vi "Reset.vi"(8 "error in (no error)":errorcluster, 11 "VISA resource name":refnum<visa-resource-name>) -> (0 "error out":errorcluster, 3 "VISA resource name out":refnum<visa-resource-name>)   [LabVIEW 2012]
doc: "Resets the instruments."
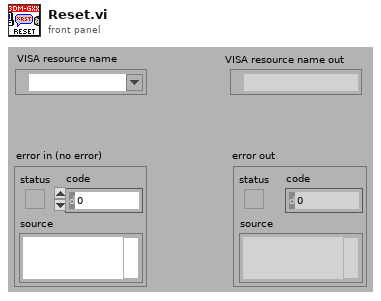
[diagram p1: front panel]
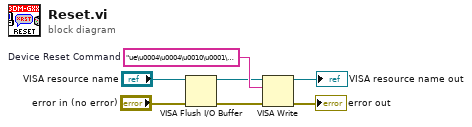
[diagram p0: block diagram]
diagram:
  w7 = "ue\u0004\u0004\u0010\u0001\u0002"  # Device Reset Command
  n1 = VISA Flush I/O Buffer(VISA resource name="VISA resource name", error in (no error)="error in (no error)") -> (VISA resource name out=w2:refnum<visa-resource-name>, error out=w1:errorcluster)  [unwired: 1 in]
  n2 = VISA Write(VISA resource name=w2, write buffer=w7, error in (no error)=w1) -> (VISA resource name out=→"VISA resource name out":refnum<visa-resource-name>, error out=→"error out":errorcluster)  [unwired: 1 out]
